vi "Self-Test.vi"(8 "error in (no error)":errorcluster, 11 "VISA resource name":refnum<visa-resource-name>) -> (0 "error out":errorcluster, 1 "Self-Test Result Message":string, 2 "Self-Test Result Code":i32, 3 "VISA resource name out":refnum<visa-resource-name>)   [LabVIEW 2013, in "Watts Up Series.lvlib"]
doc: "Runs the instrument's self-test routine and returns the test results."
uses:
  <instrlib>/Watts Up Series/Watts Up Series.lvlib
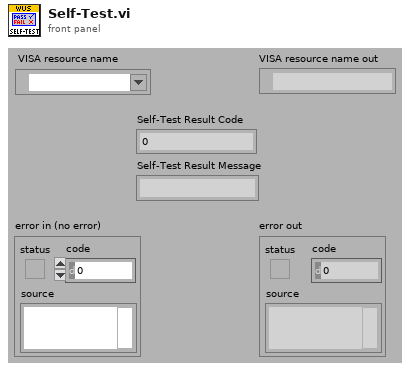
[diagram p1: front panel]
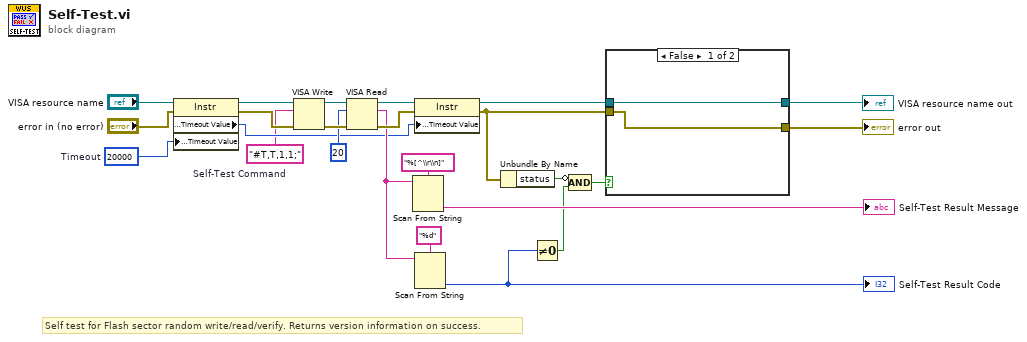
[diagram p0: block diagram]
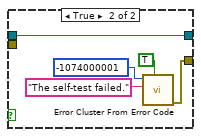
[diagram p2: hidden frame]
diagram:
  w13 = u32 20000  # Timeout
  w9 = "#T,T,1,1;"  # Self-Test Command
  # "Self test for Flash sector random write/read/verify. Returns version information on success."
  n1 = property class="Instr"(reference="VISA resource name", error in="error in (no error)", "General Settings:Timeout Value"=w13) -> (reference out=w11:refnum<visa-resource-name>, error out=w12:errorcluster, "General Settings:Timeout Value"=w10:u32)
  n2 = VISA Write(VISA resource name=w11, write buffer=w9, error in (no error)=w12) -> (VISA resource name out=w20:refnum<visa-resource-name>, error out=w19:errorcluster)  [unwired: 1 out]
  n3 = VISA Read(VISA resource name=w20, byte count=u32 20 ("byte count (20)"), error in (no error)=w19) -> (VISA resource name out=w22:refnum<visa-resource-name>, read buffer=w15:string, error out=w21:errorcluster)  [unwired: 1 out]
  n4 = Scan From String(format string="%[^\\r\\n]" ("Format String"), input string=w15) -> (output 1=→"Self-Test Result Message":string)  [unwired: 3 in, 3 out]
  n5 = property class="Instr"(reference=w22, error in=w21, "General Settings:Timeout Value"=w10) -> (reference out=w8:refnum<visa-resource-name>, error out=w7:errorcluster)
  n6 = Scan From String(format string="%d", input string=w15) -> (output 1=w3:i32)  [unwired: 3 in, 3 out]
  "Self-Test Result Code" <- w3
  n7 = Unbundle By Name(w7) -> ("status"=w5:bool)
  n8 = Not Equal To 0?(x=w3) -> (x != 0?=w6:bool)
  n9 = Compound Arithmetic op=AND(invert w5, w6) -> (w4:bool)
  n10 = case shown="False" w4 {
    tunnel: w8 -> [w26 w31]
    tunnel: w7 -> [w25 _]
    tunnel: [w25 w27] -> w1
    tunnel: [w26 w31] -> w2
    frame False {
    }
    frame True {
      n11 = call <vilib>:"Error Cluster From Error Code.vi"("show call chain? (False)"=TRUE, "error message (\"\")"="The self-test failed." ("Source (VI Name)"), "error code (0)"=-1074000001 ("Code")) -> ("error out"=w27:errorcluster)  [unwired: 6 in]
    }
  }
  "VISA resource name out" <- w2
  "error out" <- w1
